vi "Split recorder_trace block item from answer.vi"(0 "Slice block item":i32 min=1 max=4 step=1, 2 "RecorderIDs to query":string[](array[string]), 3 "TraceIDs to query":i32[](array[numeric]) min=1 max=4 step=1, 4 "Input string":string, 5 "error in":errorcluster) -> (14 "Sliced text segments":string[](array[string]), 19 "error out":errorcluster)   [LabVIEW 2020]
panel:
  # "Slice specific recorder answer into text segments."
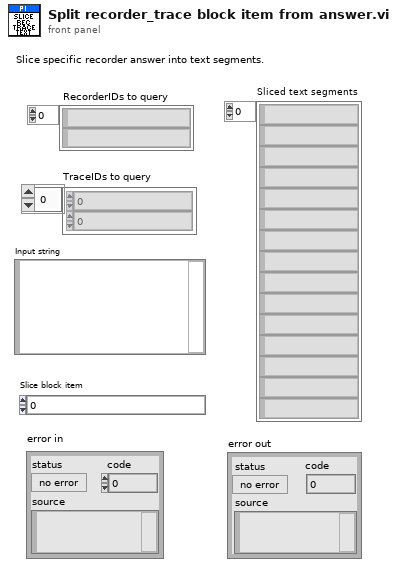
[diagram p1: front panel]
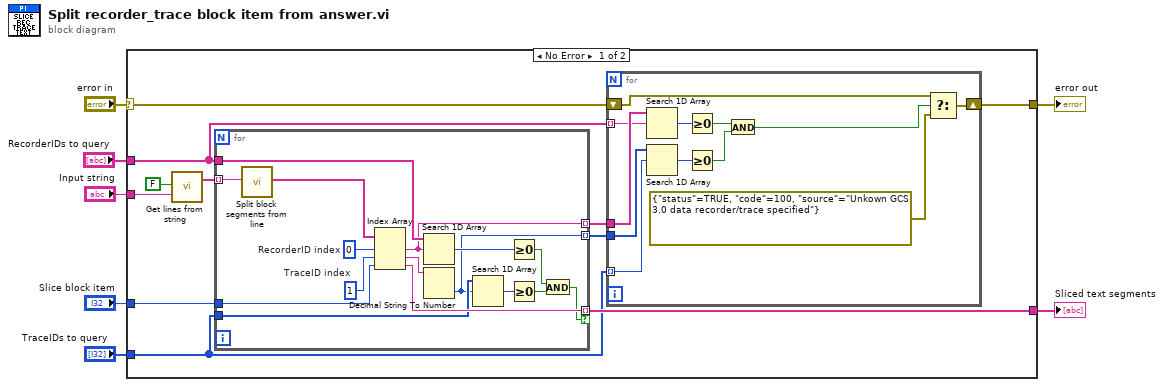
[diagram p0: block diagram]
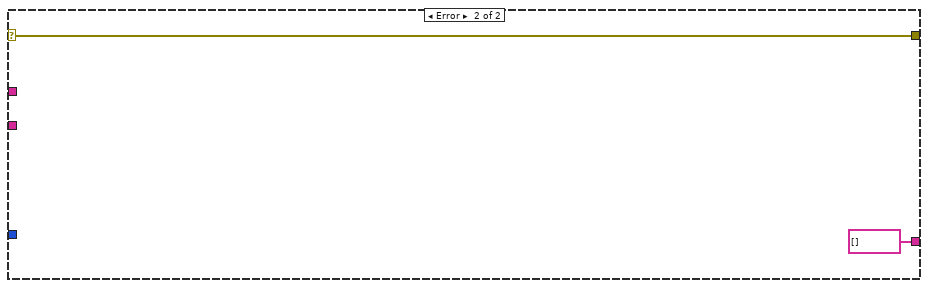
[diagram p2: hidden frame]
diagram:
  n1 = case shown="No Error" "error in" {
    selector: "error in" -> [w11 w48]
    tunnel: [w10 w48] -> w6
    tunnel: "RecorderIDs to query" -> [w13 _]
    tunnel: [w16 string[] [] ("Sliced text segments")] -> w4
    tunnel: "Slice block item" -> [w15 _]
    tunnel: "Input string" -> [w14 _]
    tunnel: "TraceIDs to query" -> [w12 _]
    frame No Error {
      n2 = call "Get lines from string.vi"("Cut spaces?"=FALSE, "Input string"=w14) -> ("Strings"=w18:string[])  [unwired: 16 in, 1 out]
      n3 = for {
        tunnel: w18 -> [w45] mode=indexing
        tunnel: w15 -> [w41]
        tunnel: [w39] -> w16 mode=indexing if=w35
        tunnel: w13 -> [w43]
        tunnel: w12 -> [w38]
        tunnel: [w33] -> w9 mode=indexing
        tunnel: [w31] -> w8 mode=indexing
        w40 = 1  # TraceID index
        w44 = 0  # RecorderID index
        n4 = call "Split block segments from line.vi"("Input line string"=w45) -> ("Text segments"=w46:string[])  [unwired: 18 in]
        n5 = Index Array(array=w46, index #1=w44, index #2=w40, index #3=w41) -> (element #1=w33:string, element #2=w32:string, element #3=w39:string)
        n6 = Search 1D Array(1D array=w43, element=w33) -> (index of element=w42:i32)  [unwired: 1 in]
        n7 = Decimal String To Number(string=w32) -> (number=w31:i32)  [unwired: 2 in, 1 out]
        n8 = Search 1D Array(1D array=w38, element=w31) -> (index of element=w34:i32)  [unwired: 1 in]
        n9 = Greater Or Equal To 0?(x=w42) -> (x >= 0?=w36:bool)
        n10 = Greater Or Equal To 0?(x=w34) -> (x >= 0?=w37:bool)
        n11 = And(x=w36, y=w37) -> (x .and. y?=w35:bool)
      }
      n12 = for {
        tunnel: w13 -> [w29] mode=indexing
        tunnel: w12 -> [w23] mode=indexing
        shift-right: [w25] -> w10
        shift-left: w11 -> [w26]
        tunnel: w9 -> [w30]
        tunnel: w8 -> [w24]
        n13 = Search 1D Array(1D array=w30, element=w29) -> (index of element=w28:i32)  [unwired: 1 in]
        n14 = Search 1D Array(1D array=w24, element=w23) -> (index of element=w22:i32)  [unwired: 1 in]
        n15 = Greater Or Equal To 0?(x=w28) -> (x >= 0?=w20:bool)
        n16 = Greater Or Equal To 0?(x=w22) -> (x >= 0?=w21:bool)
        n17 = And(x=w20, y=w21) -> (x .and. y?=w19:bool)
        n18 = Select(t=w26, s=w19, f=errorcluster {"status"=TRUE, "code"=100, "source"="Unkown GCS 3.0 data recorder/trace specified"} ("error out")) -> (s? t:f=w25:errorcluster)
      }
    }
    frame Error {
    }
  }
  "error out" <- w6
  "Sliced text segments" <- w4
